vi "SELECT USER COLUMNS.vi"(8 "Search Database Results":refnum<vi>, 9 "DATA IN":string[][](array[string]), 11 "User Column Selector":T1) -> (1 "HEADERS OUT":string[](array[string]), 3 "DATA OUT":string[][](array[string]))   [LabVIEW 2019]
uses:
  Controls/Column Names/User Column Names.ctl
  <vilib>/Utility/miscctls.llb/LVRowAndColumnTypeDef.ctl
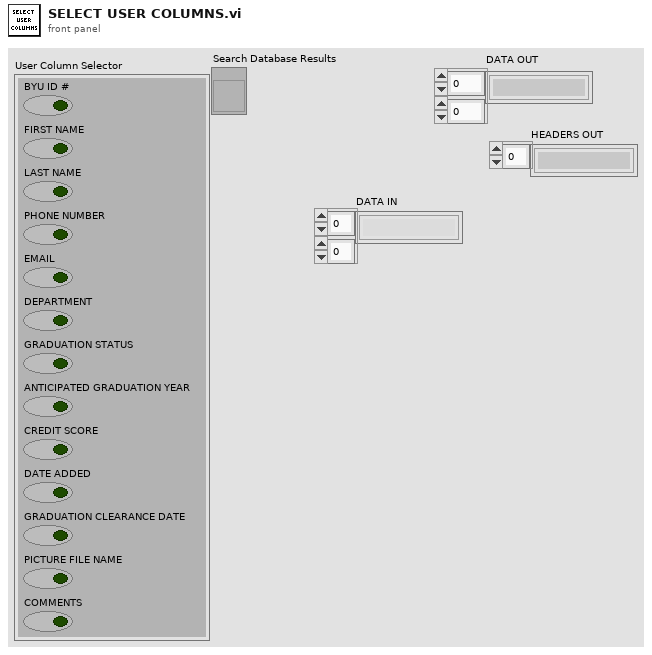
[diagram p1: front panel]
types:
  T1 = cluster{"BYU ID #":bool, "FIRST NAME":bool, "LAST NAME":bool, "PHONE NUMBER":bool, "EMAIL":bool, "DEPARTMENT":bool, "GRADUATION STATUS":bool, "ANTICIPATED GRADUATION YEAR":bool, "CREDIT SCORE":bool, "DATE ADDED":bool, "GRADUATION CLEARANCE DATE":bool, "PICTURE FILE NAME":bool, "COMMENTS":bool}
  T2 = typedef "User Column Names.ctl" = string[]
  T3 = typedef "LVRowAndColumnTypeDef.ctl" = cluster{"Row":i32, "Column":i32}
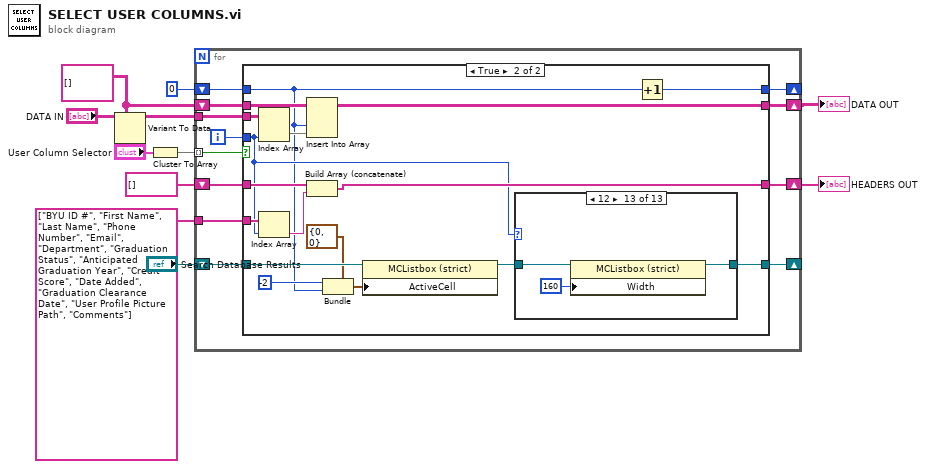
[diagram p0: block diagram]
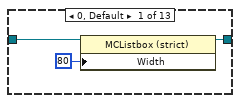
[diagram p3: hidden frame]
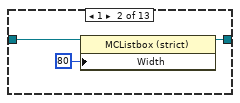
[diagram p4: hidden frame]
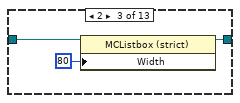
[diagram p5: hidden frame]
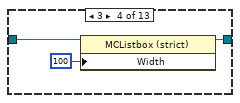
[diagram p6: hidden frame]
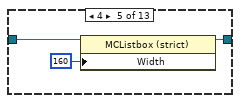
[diagram p7: hidden frame]
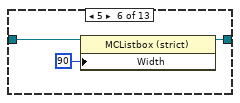
[diagram p8: hidden frame]
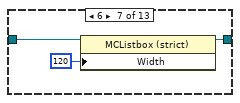
[diagram p9: hidden frame]
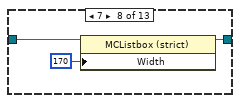
[diagram p10: hidden frame]
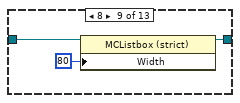
[diagram p11: hidden frame]
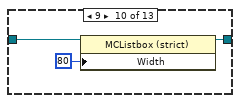
[diagram p12: hidden frame]
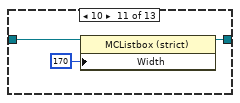
[diagram p13: hidden frame]
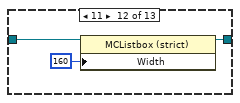
[diagram p14: hidden frame]
diagram:
  w7 = string[][] [] ("DATA OUT")
  n1 = Variant To Data(type=w7, Variant="DATA IN") -> (data=w6:string[][])  [unwired: 1 in, 1 out]
  n2 = Cluster To Array(cluster="User Column Selector") -> (array=w5:bool[])
  n3 = for {
    tunnel: w5 -> [w21] mode=indexing
    tunnel: w6 -> [w23]
    shift-right: [w17] -> w10
    shift-left: w7 -> [w20]
    shift-right: [w18] -> _
    shift-left: 0 -> [w19]
    tunnel: T2 ["BYU ID #", "First Name", "Last Name", "Phone Number", "Email", "Department", "Graduation Status", "Anticipated Graduation Year", "Credit Score", "Date Added", "Graduation Clearance Date", "User Profile Picture Path", "Comments"] ("USER COLUMN NAMES") -> [w16]
    shift-right: [w14] -> w9
    shift-left: string[] [] ("DATA OUT") -> [w15]
    shift-right: [w12] -> _
    shift-left: "Search Database Results" -> [w13]
    i -> [w22]
    n4 = case shown="True" w21 {
      tunnel: w23 -> [_ w44]
      tunnel: w22 -> [_ w35]
      tunnel: w20 -> [w26 w43]
      tunnel: w19 -> [w27 w29]
      tunnel: [w27 w41] -> w18
      tunnel: [w26 w40] -> w17
      tunnel: w16 -> [_ w39]
      tunnel: w15 -> [w25 w38]
      tunnel: [w25 w36] -> w14
      tunnel: w13 -> [w24 w34]
      tunnel: [w24 w28] -> w12
      frame False {
      }
      frame True {
        n5 = Index Array(array=w44, index (col)=w35) -> (element=w42:string[])  [unwired: 1 in]
        n6 = Index Array(array=w39, index=w35) -> (element=w37:string)
        n7 = Insert Into Array(array=w43, index (col)=w29, new element=w42) -> (w40:string[][])  [unwired: 1 in]
        n8 = Build Array (concatenate)(w38, w37) -> (w36:string[])
        n9 = Bundle(cluster=T3 {"Row"=0, "Column"=0} ("Active Cell:Active Cell"), "Row"=-2, "Column"=w29) -> (w31:T3)
        n10 = property class="MCListbox (strict)"(reference=w34, "ActiveCell"=w31) -> (reference out=w33:refnum<vi>)  [unwired: 1 in, 1 out]
        n11 = case shown="12" w35 {
          tunnel: w33 -> [w47 w50 w53 w56 w59 w62 w65 w68 w71 w74 w77 w80 w82]
          tunnel: [w46 w49 w52 w55 w58 w61 w64 w67 w70 w73 w76 w79 w81] -> w28
          frame 0, Default {
            n12 = property class="MCListbox (strict)"(reference=w47, "Width"=u32 80 ("Active Cell:Cell Size:Width")) -> (reference out=w46:refnum<vi>)  [unwired: 1 in, 1 out]
          }
          frame 1 {
            n13 = property class="MCListbox (strict)"(reference=w50, "Width"=u32 80 ("Active Cell:Cell Size:Width")) -> (reference out=w49:refnum<vi>)  [unwired: 1 in, 1 out]
          }
          frame 2 {
            n14 = property class="MCListbox (strict)"(reference=w53, "Width"=u32 80 ("Active Cell:Cell Size:Width")) -> (reference out=w52:refnum<vi>)  [unwired: 1 in, 1 out]
          }
          frame 3 {
            n15 = property class="MCListbox (strict)"(reference=w56, "Width"=u32 100 ("Active Cell:Cell Size:Width")) -> (reference out=w55:refnum<vi>)  [unwired: 1 in, 1 out]
          }
          frame 4 {
            n16 = property class="MCListbox (strict)"(reference=w59, "Width"=u32 160 ("Active Cell:Cell Size:Width")) -> (reference out=w58:refnum<vi>)  [unwired: 1 in, 1 out]
          }
          frame 5 {
            n17 = property class="MCListbox (strict)"(reference=w62, "Width"=u32 90 ("Active Cell:Cell Size:Width")) -> (reference out=w61:refnum<vi>)  [unwired: 1 in, 1 out]
          }
          frame 6 {
            n18 = property class="MCListbox (strict)"(reference=w65, "Width"=u32 120 ("Active Cell:Cell Size:Width")) -> (reference out=w64:refnum<vi>)  [unwired: 1 in, 1 out]
          }
          frame 7 {
            n19 = property class="MCListbox (strict)"(reference=w68, "Width"=u32 170 ("Active Cell:Cell Size:Width")) -> (reference out=w67:refnum<vi>)  [unwired: 1 in, 1 out]
          }
          frame 8 {
            n20 = property class="MCListbox (strict)"(reference=w71, "Width"=u32 80 ("Active Cell:Cell Size:Width")) -> (reference out=w70:refnum<vi>)  [unwired: 1 in, 1 out]
          }
          frame 9 {
            n21 = property class="MCListbox (strict)"(reference=w74, "Width"=u32 80 ("Active Cell:Cell Size:Width")) -> (reference out=w73:refnum<vi>)  [unwired: 1 in, 1 out]
          }
          frame 10 {
            n22 = property class="MCListbox (strict)"(reference=w77, "Width"=u32 170 ("Active Cell:Cell Size:Width")) -> (reference out=w76:refnum<vi>)  [unwired: 1 in, 1 out]
          }
          frame 11 {
            n23 = property class="MCListbox (strict)"(reference=w80, "Width"=u32 160 ("Active Cell:Cell Size:Width")) -> (reference out=w79:refnum<vi>)  [unwired: 1 in, 1 out]
          }
          frame 12 {
            n24 = property class="MCListbox (strict)"(reference=w82, "Width"=u32 160 ("Active Cell:Cell Size:Width")) -> (reference out=w81:refnum<vi>)  [unwired: 1 in, 1 out]
          }
        }
        n25 = Increment(x=w29) -> (x+1=w41:i32)
      }
    }
  }
  "DATA OUT" <- w10
  "HEADERS OUT" <- w9
